vi "Wait with references.vi"(7 "seconds to wait (1)":dbl=1.0, 8 "error in (no error)":errorcluster, 11 "Common properties":T1) -> (0 "error out":errorcluster)   [LabVIEW 2020]
doc: "Wait for specified seconds, skips if error. Takes references from Common properties and reacts to Abort buttons, shows proper message etc."
uses:
  Type definitions/Common properties.ctl
  external libraries/varilib/varilib.lvlib
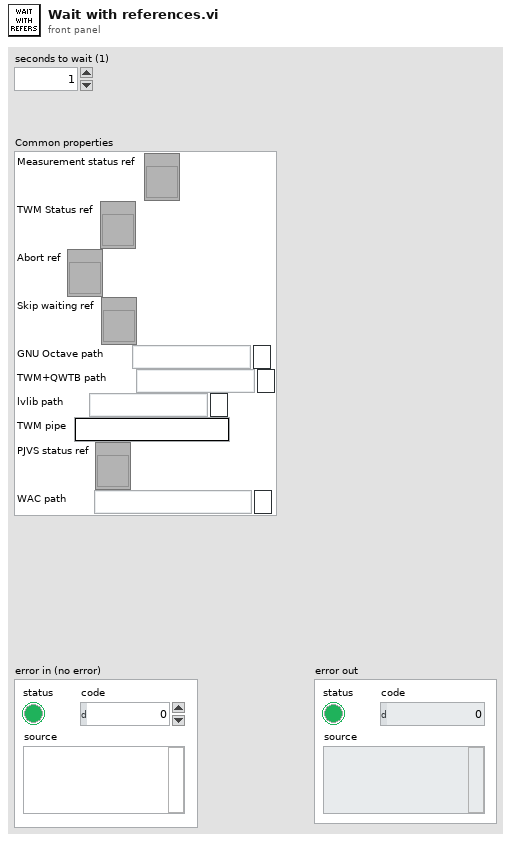
[diagram p1: front panel]
types:
  T1 = typedef "Common properties.ctl" = cluster{"Measurement status ref":refnum<vi>, "TWM Status ref":refnum<vi>, "Abort ref":refnum<vi>, "Skip waiting ref":refnum<vi>, "GNU Octave path":path, "TWM+QWTB path":path, "lvlib path":path, "TWM pipe":string, "PJVS status ref":refnum<vi>, "WAC path":path}
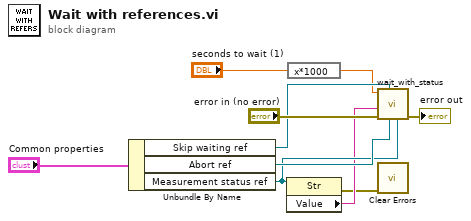
[diagram p0: block diagram]
diagram:
  n1 = Unbundle By Name("Common properties") -> ("Skip waiting ref"=w8:refnum<vi>, "Abort ref"=w9:refnum<vi>, "Measurement status ref"=w3:refnum<vi>)
  n2 = property class="Str"(reference=w3) -> (error out=w1:errorcluster, "Value"=w2:string)  [unwired: 1 in, 1 out]
  n3 = expression code="x*1000"("seconds to wait (1)") -> (w5:dbl)
  n4 = call "wait_with_status.vi"("stat ref"=w3, "stop ref"=w9, "second stop ref"=w8, "error in"="error in (no error)", "comment"=w2, "ms to wait"=w5) -> ("error out"=→"error out":errorcluster)  [unwired: 4 in, 1 out]
  n5 = call <vilib>:"Clear Errors.vi"("error in (no error)"=w1) -> ()  [unwired: 5 in, 2 out]
